vi "acquire single wave init subvi.vi"(10 "Enum in":enum16{"Idle", "Start"}(ring), 11 "VISA Refnum in":refnum<visa-resource-name>="USB0::0x5345::0x1234::SERIAL::RAW") -> (0 "error out":errorcluster, 1 "read buffer":string, 2 "Enum out":enum16{"Idle", "Start"}(ring), 3 "VISA Refnum out":refnum<visa-resource-name>)   [LabVIEW 2013]
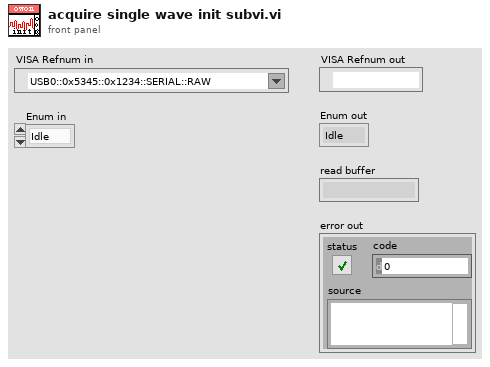
[diagram p1: front panel]
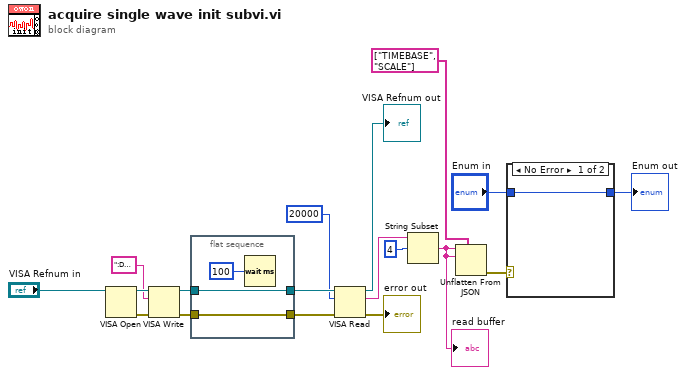
[diagram p0: block diagram]
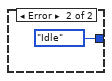
[diagram p2: hidden frame]
diagram:
  n1 = VISA Open(VISA resource name="VISA Refnum in") -> (VISA resource name=w9:refnum<visa-resource-name>, error out=w10:errorcluster)  [unwired: 4 in]
  n2 = VISA Write(VISA resource name=w9, write buffer=":DATA:WAVE:SCREEN:HEAD?" ("ID Query"), error in (no error)=w10) -> (VISA resource name out=w16:refnum<visa-resource-name>, error out=w18:errorcluster)  [unwired: 1 out]
  n3 = flat-sequence {
    tunnel: [w21] -> w15
    tunnel: w16 -> [w21]
    tunnel: [w20] -> w17
    tunnel: w18 -> [w20]
    frame #0 {
      n4 = Wait (ms)(milliseconds to wait=u32 100 ("等待时间（毫秒）")) -> ()  [unwired: 1 out]
    }
  }
  n5 = VISA Read(VISA resource name=w15, byte count=u32 20000, error in (no error)=w17) -> (VISA resource name out=→"VISA Refnum out":refnum<visa-resource-name>, read buffer=w6:string, error out=→"error out":errorcluster)  [unwired: 1 out]
  n6 = String Subset(string=w6, offset (0)=4) -> (substring=w13:string)  [unwired: 1 in]
  "read buffer" <- w13
  n7 = Unflatten From JSON(path=string[] ["TIMEBASE", "SCALE"], JSON string=w13, type and defaults=w13) -> (error out=w14:errorcluster)  [unwired: 4 in, 1 out]
  n8 = case shown="No Error" w14 {
    tunnel: [w22 enum16{"Idle", "Start"}."Idle"] -> w11
    tunnel: "Enum in" -> [w22 _]
    frame No Error {
    }
    frame Error {
    }
  }
  "Enum out" <- w11
